vi "OAT Form Orders String.vi"(1 "orders to extract in":dbl[](array[numeric])=[1.0]) -> (0 "orders to extract out":string="Order 1.0")   [LabVIEW 2017, in "SoundVib_Gabor.lvlib"]
uses:
  <vilib>/addons/Sound and Vibration/Order Analysis/Gabor Order Tracking/SoundVib_Gabor.lvlib
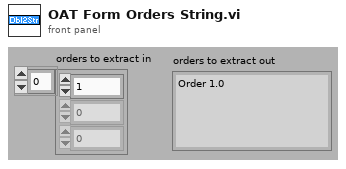
[diagram p1: front panel]
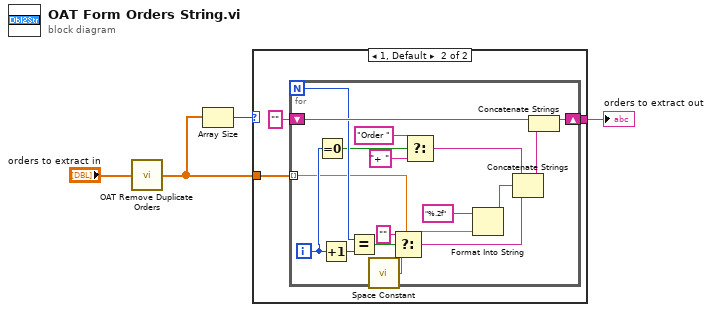
[diagram p0: block diagram]
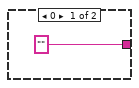
[diagram p2: hidden frame]
diagram:
  n1 = call <vilib>:"OAT Remove Duplicate Orders.vi"("array in"="orders to extract in") -> ("array out"=w1:dbl[])
  n2 = Array Size(array=w1) -> (size(s)=w4:i32)
  n3 = case shown="1, Default" w4 {
    tunnel: w1 -> [_ w8]
    tunnel: ["" ("Orders to extract out") w6] -> w3
    frame 0 {
    }
    frame 1, Default {
      n4 = for {
        N -> [w21]
        tunnel: w8 -> [w11] mode=indexing
        shift-right: [w24] -> w6
        shift-left: "" ("Orders to extract out") -> [w25]
        i -> [w17]
        n5 = Equal To 0?(x=w17) -> (x = 0?=w16:bool)
        n6 = Increment(x=w17) -> (x+1=w22:i32)
        n7 = Equal?(x=w21, y=w22) -> (x = y?=w20:bool)
        n8 = call <vilib>:"Space Constant.vi"() -> ("String"=w12:string)
        n9 = Select(t="" ("Orders to extract out"), s=w20, f=w12) -> (s? t:f=w18:string)
        n10 = Select(t="Order " ("Substring"), s=w16, f="+ " ("Orders to extract out")) -> (s? t:f=w13:string)
        n11 = Format Into String(format string="%.2f", w11) -> (resulting string=w10:string)  [unwired: 2 in, 1 out]
        n12 = Concatenate Strings(w13, w10, w18) -> (w23:string)
        n13 = Concatenate Strings(w25, w23) -> (w24:string)
      }
    }
  }
  "orders to extract out" <- w3
